vi "UHR-Fleezers Control (host) - 12.0.vi"() -> ()   [LabVIEW 2012] (continued)
                n291 = Divide "X half step offset"(x=w508, y=2.0) -> (x/y=w516:dbl)
                n292 = Divide "X V/pix"(x=w508, y=w519) -> (x/y=w518:dbl)
                n293 = Multiply(x=w508, y=w513) -> (x*y=w525:dbl)
                n294 = Compound Arithmetic op=ADD(w523, w530, w529) -> (w500:dbl)
                "Pointer Y (V)" <- w500
                n295 = Multiply(x=w518, y=w512) -> (x*y=w527:dbl)
                n296 = Negate(x=w516) -> (-x=w515:dbl)
                n297 = local read "Initial X"() -> (w528:dbl)
                n298 = Negate(x=w527) -> (-x=w526:dbl)
                n299 = Compound Arithmetic op=ADD(w515, w525, w528, w526) -> (w501:dbl)
                "Pointer X (V)" <- w501
                n300 = case shown="True" "Set High F Confocal Spot (X-Y)" {
                  tunnel: w501 -> [_ w531]
                  tunnel: w500 -> [_ w532]
                  frame False {
                  }
                  frame True {
                    "Confocal Y 2 (V)" <- w532
                    "Confocal X 2 (V)" <- w531
                  }
                }
                n301 = Or(x="Set X Only", y="Set Confocal Spot (X-Y)") -> (x .or. y?=w504:bool)
                n302 = Or(x="Set Confocal Spot (X-Y)", y="Set Y Only") -> (x .or. y?=w503:bool)
                n303 = case shown="True" w504 {
                  tunnel: w501 -> [_ w533]
                  frame False {
                  }
                  frame True {
                    n304 = property on="AO2" class="Slide (strict)"("Val(Sgnl)"=w533) -> ()  [unwired: 2 in, 2 out]
                    "Confocal X 1 (V)" <- w533
                  }
                }
                n305 = case shown="True" w503 {
                  tunnel: w500 -> [_ w534]
                  frame False {
                  }
                  frame True {
                    n306 = property on="AO1" class="Slide (strict)"("Val(Sgnl)"=w534) -> ()  [unwired: 2 in, 2 out]
                    "Confocal Y 1 (V)" <- w534
                  }
                }
                n307 = local write "Set High F Confocal Spot (X-Y)"(w499) -> ()
                n308 = local write "Set Confocal Spot (X-Y)"(w499) -> ()
                n309 = local write "Set X Only"(w499) -> ()
                n310 = local write "Set Y Only"(w499) -> ()
              }
            }
          }
          frame 3 {
            n311 = local read "BD 2 Frequency 1 (MHz)"() -> (w535:dbl)
            n312 = local read "BD 1 Frequency 1 (MHz)"() -> (w536:dbl)
            n313 = local write "Manipulating Trap"(TRUE ("Manipulating Trap")) -> ()
            n314 = local write "Coords"(T7 {"Horizontal"=0, "Vertical"=0} ("Coords")) -> ()
            n315 = while {
              tunnel: w541 -> [w546]
              tunnel: w539 -> [w545]
              tunnel: w537 -> [w544]
              tunnel: w536 -> [w543]
              tunnel: w535 -> [w542]
              stop <- w547 stop-if-true
              n316 = event shown="[0] \"Pane\": Mouse Move" {
                selector: _ -> [_ _]
                dyn-events: _ -> [_ _]
                timeout: _ -> [_ _]
                tunnel: ["Force Manip Abort" w611] -> w547
                tunnel: w546 -> [w554 _]
                tunnel: w545 -> [w552 _]
                tunnel: w544 -> [w551 _]
                tunnel: w543 -> [w550 _]
                tunnel: w542 -> [w549 _]
                event Mouse Move {
                  n317 = event-data() -> ("Time"=w555:u32, "Coords"=w556:T7)  [unwired: 3 out]
                  n318 = Less?(x=w555, y=w554) -> (x < y?=w553:bool)
                  n319 = case "Makes sure old motion events prior to mouse click aren't used" shown="False" w553 {
                    tunnel: w556 -> [w598 _]
                    tunnel: w552 -> [w599 _]
                    tunnel: w551 -> [w576 _]
                    tunnel: w550 -> [w572 _]
                    tunnel: w549 -> [w571 _]
                    frame False {
                      n320 = Subtract(x=w598, y=w599) -> (x-y=w597:T7)
                      "Coords" <- w597
                      n321 = local read "Y RF Frequency Limits (MHz)"() -> (w557:T16)
                      n322 = To Double Precision Float(number=w597) -> (double precision float=w596:cluster{"Horizontal":dbl, "Vertical":dbl})
                      n323 = Multiply(x=cluster{"Horizontal":dbl, "Vertical":dbl} {"Horizontal"=-1.0, "Vertical"=1.0}, y="Manipulation Scaling") -> (x*y=w592:cluster{"Horizontal":dbl, "Vertical":dbl})
                      n324 = local read "X RF Frequency Limits (MHz)"() -> (w558:T16)
                      n325 = Multiply(x=w596, y=w592) -> (x*y=w594:cluster{"Horizontal":dbl, "Vertical":dbl})
                      n326 = Unbundle By Name(w594) -> ("Horizontal"=w589:dbl, "Vertical"=w593:dbl)
                      n327 = Unbundle By Name(w557) -> ("Maximum"=w560:dbl, "Minimum"=w559:dbl)
                      n328 = Boolean To (0,1)(Boolean="Manip. X?") -> (0, 1=w587:i16)
                      n329 = Boolean To (0,1)(Boolean="Manip. Y?") -> (0, 1=w584:i16)
                      n330 = local read "BD 1 Frequency 2 (MHz)"() -> (w574:dbl)
                      n331 = Multiply(x=w593, y=w584) -> (x*y=w586:dbl)
                      n332 = Multiply(x=w587, y=w589) -> (x*y=w590:dbl)
                      n333 = local read "BD 2 Frequency 2 (MHz)"() -> (w573:dbl)
                      n334 = Unbundle By Name(w558) -> ("Maximum"=w562:dbl, "Minimum"=w561:dbl)
                      n335 = Add(x=w571, y=w586) -> (x+y=w564:dbl)
                      n336 = Add(x=w572, y=w590) -> (x+y=w566:dbl)
                      n337 = In Range and Coerce(upper limit=w562, x=w566, lower limit=w561) -> (coerced(x)=w565:dbl)  [unwired: 1 out]
                      n338 = In Range and Coerce(upper limit=w560, x=w564, lower limit=w559) -> (coerced(x)=w563:dbl)  [unwired: 1 out]
                      n339 = Subtract(x=w565, y=w574) -> (x-y=w583:dbl)
                      n340 = Subtract(x=w563, y=w573) -> (x-y=w582:dbl)
                      n341 = Square(x=w583) -> (x^2=w581:dbl)
                      n342 = Square(x=w582) -> (x^2=w580:dbl)
                      n343 = Add(x=w581, y=w580) -> (x+y=w579:dbl)
                      n344 = Square Root(x=w579) -> (sqrt(x)=w575:dbl)
                      n345 = In Range and Coerce(upper limit="Limit Max (MHz)", x=w575, lower limit="Limit Min (MHz)") -> (In Range?=w568:bool)  [unwired: 1 out]
                      n346 = Not(x="Limits Enable") -> (.not. x?=w567:bool)
                      n347 = Or(x=w568, y=w567) -> (x .or. y?=w569:bool)
                      n348 = case shown="True" w569 {
                        tunnel: w576 -> [_ w609]
                        tunnel: w575 -> [_ w600]
                        tunnel: w565 -> [_ w607]
                        tunnel: w574 -> [_ w606]
                        tunnel: w563 -> [_ w605]
                        tunnel: w573 -> [_ w604]
                        tunnel: w558 -> [_ w602]
                        tunnel: w557 -> [_ w601]
                        frame False {
                        }
                        frame True {
                          n349 = local read "BD 1 Frequency 3 (MHz)"() -> (w608:dbl)
                          n350 = local read "BD 2 Frequency 3 (MHz)"() -> (w603:dbl)
                          n351 = local write "Trap Delta (MHz)"(w600) -> ()
                          n352 = call "set RF board frequency - interlace.vi"("Board 2 Frequency Limits"=w601, "Board 1 Frequency Limits"=w602, "FPGA VI Reference In"=w609, "Board 2 Frequency 3 (MHz)"=w603, "Board 1 Frequency 3 (MHz)"=w608, "Board 2 Frequency 2 (MHz)"=w604, "Board 2 Frequency 1 (MHz)"=w605, "Board 1 Frequency 2 (MHz)"=w606, "Board 1 Frequency 1  (MHz)"=w607) -> ()  [unwired: 1 in, 2 out]
                          n353 = local write "BD 2 Frequency 1 (MHz)"(w605) -> ()
                          n354 = local write "BD 1 Frequency 1 (MHz)"(w607) -> ()
                        }
                      }
                    }
                    frame True {
                    }
                  }
                }
                event Mouse Up {
                  n355 = event-data() -> ("Button"=w610:u16)  [unwired: 8 out]
                  n356 = case shown="3" w610 {
                    tunnel: [FALSE TRUE] -> w611
                    frame 0, Default {
                    }
                    frame 3 {
                      n357 = local read "Trap Delta (MHz)"() -> (w613:dbl)
                      n358 = property on="Initial delta (MHz)" class="DigNum (strict)"("Val(Sgnl)"=w613) -> ()  [unwired: 2 in, 2 out]
                      n359 = local write "Manipulating Trap"(FALSE ("Manipulating Trap")) -> ()
                    }
                  }
                }
              }
            }
          }
        }
      }
      event Mouse Move {
        n360 = event-data() -> ()  [unwired: 6 out]
      }
    }
    n361 = local read "Stop All"() -> (w429:bool)
    n362 = node-c288() -> ()  [unwired: 2 out]
  }
  n363 = timed-loop "Run Scripts, including: stage motion" {
    tunnel: w89 -> [w622]
    tunnel: w88 -> [w623]
    tunnel: [w623] -> w87
    tunnel: [w622] -> w86
    timing: w84 -> [_]
    timing-out: [_] -> w83
    tunnel: w69 -> [w621]
    tunnel: w70 -> [w620]
    tunnel: w10 -> [w617]
    tunnel: w9 -> [w616]
    tunnel: w8 -> [w618]
    tunnel: w7 -> [w619]
    stop <- w624 stop-if-true
    n364 = node-c288() -> ()  [unwired: 1 in, 1 out]
    n365 = event shown="[12] \"Force FB Data Script\": Value Change" {
      selector: _ -> [_ _ _ _ _ _ _ _ _ _ _ _ _ _ _ _ _ _ _]
      dyn-events: _ -> [_ _ _ _ _ _ _ _ _ _ _ _ _ _ _ _ _ _ _]
      timeout: _ -> [_ _ _ _ _ _ _ _ _ _ _ _ _ _ _ _ _ _ _]
      tunnel: ["Set Position" "Move to Position" _ _ "Read Harvard" _ _ _ _ _ _ "Got ADig bead" "Force FB Data\nScript" _ "Got DNA bead" "Take Stepping Data" _ "Take Detection Laser\nImage" _] -> _
      tunnel: [_ _ _ _ _ _ _ _ _ _ _ _ _ _ _ _ _ _ w1241] -> w624
      tunnel: w622 -> [w642 w650 w663 w693 _ w738 w778 w859 w888 w1020 w1046 _ w1082 _ _ _ _ _ _]
      tunnel: w623 -> [w643 w651 w664 w694 _ w739 w779 w860 w889 w1021 w1047 _ w1083 _ _ _ _ _ _]
      tunnel: w621 -> [_ _ _ _ w723 _ _ _ _ _ _ _ _ _ _ _ _ _ _]
      tunnel: w620 -> [_ _ _ _ w722 _ _ _ _ _ _ _ _ _ _ _ _ _ _]
      tunnel: w619 -> [_ _ _ _ _ _ _ _ _ _ _ _ _ _ _ _ _ _ _]
      tunnel: w618 -> [_ _ _ _ _ _ _ _ _ _ _ _ _ _ _ _ _ _ _]
      tunnel: w617 -> [_ _ _ _ _ _ _ _ _ _ _ _ _ _ _ _ _ _ _]
      tunnel: w616 -> [_ _ _ _ _ _ _ _ _ _ _ _ _ _ _ _ _ _ _]
      event "Set Position", "Set Position 2", "Set Position 3", "Set Position 4", "Set Position 5", "Set Position 1": Value Change {
        n366 = event-data() -> ()  [unwired: 1 in, 5 out]
        n367 = Build Array("Set Position 1", "Set Position 2", "Set Position 3", "Set Position 4", "Set Position 5") -> (w641:bool[])
        n368 = Boolean Array To Number(Boolean array=w641) -> (number=w640:u32)
        n369 = Logarithm Base 2(1:w640) -> (0:w632:dbl)
        n370 = call "Read Stage Position.vi"("error in"=w642, "VISA resource name in"=w643) -> ("Current Position"=w647:cluster{dbl, dbl, dbl}, "error out"=w646:errorcluster)  [unwired: 2 out]
        n371 = Decrement(x="Position") -> (x-1=w630:dbl)
        n372 = Greater Or Equal?(x=w632, y=0.0) -> (x >= y?=w633:bool)
        n373 = Cluster To Array(cluster=w647) -> (array=w644:dbl[])
        n374 = local write "Stage Control Serial Error"(w646) -> ()
        n375 = Select(t=w632, s=w633, f=w630) -> (s? t:f=w629:dbl)
        n376 = Increment(x=w629) -> (x+1=w628:dbl)
        n377 = Build Array (concatenate)(w628, w644) -> (w627:dbl[])
        n378 = Replace Array Subset(array="Saved Stage Positions", new element=w627, index (row)=w629) -> (w645:dbl[][])  [unwired: 1 in]
        n379 = local write "Saved Stage Positions"(w645) -> ()
      }
      event "Move to Position": Value Change {
        n380 = event-data() -> ()  [unwired: 1 in, 5 out]
        n381 = flat-sequence {
          tunnel: w651 -> [w655]
          tunnel: w650 -> [w654]
          frame #0 {
            n382 = local read "Saved Stage Positions"() -> (w657:dbl[][])
            n383 = local read "Position"() -> (w656:dbl)
            n384 = local write "Stage Moving"(TRUE ("Stage Moving")) -> ()
            n385 = call "move to saved stage position.vi"("error in"=w654, "Stage VISA resource name in"=w655, "Position"=w656, "Saved Stage Positions"=w657) -> ("error out"=w653:errorcluster)  [unwired: 1 out]
            n386 = local write "Stage Control Serial Error"(w653) -> ()
          }
          frame #1 {
            n387 = call <vilib>:"Beep.vi"() -> ()  [unwired: 3 in, 9 out]
            n388 = local write "Stage Moving"(FALSE ("Stage Moving")) -> ()
          }
        }
      }
      event "Move Cap. 1 (DNA Bottom)": Value Change {
        n389 = event-data() -> ()  [unwired: 1 in, 5 out]
        n390 = local write "Move Cap. 1 (DNA Bottom)"(FALSE ("Move Cap. 1 (DNA Right)")) -> ()
        n391 = flat-sequence {
          tunnel: w663 -> [w666]
          tunnel: w664 -> [w667]
          tunnel: [w667] -> w661
          tunnel: [w666] -> w660
          tunnel: w661 -> [w669]
          tunnel: w660 -> [w668]
          frame #0 {
            n392 = property on="Sample Channel\nFlow" class="Bool (strict)"("Val(Sgnl)"="Cap 1 Samp Flow ON") -> ()  [unwired: 2 in, 2 out]
          }
          frame #1 {
            n393 = local read "Saved Stage Positions"() -> (w679:dbl[][])
            n394 = local write "Stage Moving"(TRUE ("Stage Moving")) -> ()
            n395 = Array Subset(array=w679, index (row)=0 ("index"), length (row)=1 ("length"), index (col)=1 ("index"), length (col)=3 ("length")) -> (w676:dbl[][])
            n396 = Reshape Array(w676, 3 ("dimension size")) -> (w674:dbl[])
            n397 = Array To Cluster(array=w674) -> (cluster=w673:cluster{"[0]":dbl, "[1]":dbl, "[2]":dbl})
            n398 = call "Set Stage Position.vi"("Position"=w673, "error in"=w668, "VISA resource name in"=w669) -> ("error out"=w672:errorcluster)  [unwired: 2 out]
            n399 = local write "Stage Control Serial Error"(w672) -> ()
          }
          frame #2 {
            n400 = local write "Stage Moving"(FALSE ("Stage Moving")) -> ()
            n401 = case shown="True" "Cap 1 Flow ON" {
              frame False {
              }
              frame True {
                n402 = property on="Inject Pump 1" class="Bool (strict)"("Val(Sgnl)"=TRUE ("Value (Signaling)")) -> ()  [unwired: 2 in, 2 out]
              }
            }
            n403 = call <vilib>:"Beep.vi"() -> ()  [unwired: 3 in, 9 out]
          }
          frame #3 {
            n404 = property on="Sample Channel\nFlow" class="Bool (strict)"("Val(Sgnl)"=FALSE ("Value (Signaling)")) -> ()  [unwired: 2 in, 2 out]
            n405 = local read "Cap. 2 BD T1?\n(ADig T1, DNA T2)"() -> (w686:bool)
            n406 = case shown="True" w686 {
              tunnel: "Cap 1 T ON" -> [w688 w689]
              frame False {
                n407 = property on="Trap 1 (ON/OFF)" class="Bool (strict)"("Val(Sgnl)"=w688) -> ()  [unwired: 2 in, 2 out]
              }
              frame True {
                n408 = property on="Trap 2 (ON/OFF)" class="Bool (strict)"("Val(Sgnl)"=w689) -> ()  [unwired: 2 in, 2 out]
              }
            }
            n409 = property on="Got DNA bead" class="Bool"("Key Focus"=TRUE) -> ()  [unwired: 2 in, 2 out]
          }
        }
      }
      event "Move Cap. 2 (ADig Top)": Value Change {
        n410 = event-data() -> ()  [unwired: 1 in, 5 out]
        n411 = local write "Move Cap. 2 (ADig Top)"(FALSE ("Move Cap. 2 (ADig Left)")) -> ()
        n412 = flat-sequence {
          tunnel: w693 -> [w696]
          tunnel: w694 -> [w697]
          tunnel: [w697] -> w691
          tunnel: [w696] -> w690
          tunnel: w691 -> [w700]
          tunnel: w690 -> [w699]
          frame #0 {
            n413 = property on="Sample Channel\nFlow" class="Bool (strict)"("Val(Sgnl)"="Cap 2 Samp Flow ON") -> ()  [unwired: 2 in, 2 out]
          }
          frame #1 {
            w698 = FALSE ("Value (Signaling)")
            n414 = local read "Saved Stage Positions"() -> (w710:dbl[][])
            n415 = local write "Stage Moving"(TRUE ("Stage Moving")) -> ()
            n416 = Array Subset(array=w710, index (row)=1 ("index"), length (row)=1 ("length"), index (col)=1 ("index"), length (col)=3 ("length")) -> (w707:dbl[][])
            n417 = Reshape Array(w707, 3 ("dimension size")) -> (w705:dbl[])
            n418 = property on="Trap 1 (ON/OFF)" class="Bool (strict)"("Val(Sgnl)"=w698) -> ()  [unwired: 2 in, 2 out]
            n419 = property on="Trap 1 (ON/OFF)" class="Bool (strict)"("Val(Sgnl)"=w698) -> ()  [unwired: 2 in, 2 out]
            n420 = Array To Cluster(array=w705) -> (cluster=w704:cluster{"[0]":dbl, "[1]":dbl, "[2]":dbl})
            n421 = call "Set Stage Position.vi"("Position"=w704, "error in"=w699, "VISA resource name in"=w700) -> ("error out"=w703:errorcluster)  [unwired: 2 out]
            n422 = local write "Stage Control Serial Error"(w703) -> ()
          }
          frame #2 {
            n423 = local write "Stage Moving"(FALSE ("Stage Moving")) -> ()
            n424 = call <vilib>:"Beep.vi"() -> ()  [unwired: 3 in, 9 out]
            n425 = case shown="True" "Cap 2 Flow ON" {
              frame False {
              }
              frame True {
                n426 = property on="Inject Pump 3" class="Bool (strict)"("Val(Sgnl)"=TRUE ("Value (Signaling)")) -> ()  [unwired: 2 in, 2 out]
              }
            }
          }
          frame #3 {
            n427 = property on="Sample Channel\nFlow" class="Bool (strict)"("Val(Sgnl)"=FALSE ("Value (Signaling)")) -> ()  [unwired: 2 in, 2 out]
            n428 = case shown="False" "Cap. 2 BD T1?\n(ADig T1, DNA T2)" {
              tunnel: "Cap 2 T ON" -> [w719 w720]
              frame False {
                n429 = property on="Trap 2 (ON/OFF)" class="Bool (strict)"("Val(Sgnl)"=w719) -> ()  [unwired: 2 in, 2 out]
              }
              frame True {
                n430 = property on="Trap 1 (ON/OFF)" class="Bool (strict)"("Val(Sgnl)"=w720) -> ()  [unwired: 2 in, 2 out]
              }
            }
            n431 = property on="Got ADig bead" class="Bool"("Key Focus"=TRUE) -> ()  [unwired: 2 in, 2 out]
          }
        }
      }
      event "Read Harvard": Value Change {
        n432 = event-data() -> ()  [unwired: 1 in, 5 out]
        n433 = Concatenate Strings("write buffer", "\r") -> (w725:string)
        n434 = VISA Write(VISA resource name=w723, write buffer=w725, error in (no error)=w722) -> (VISA resource name out=w734:refnum<visa-resource-name>, error out=w733:errorcluster)  [unwired: 1 out]
        n435 = stacked-sequence {
          tunnel: [w737] -> w732
          tunnel: w734 -> [w737]
          tunnel: w733 -> [w736]
          tunnel: [w736] -> w727
          frame #0 {
            n436 = Wait (ms)(milliseconds to wait=50) -> ()  [unwired: 1 out]
          }
        }
        n437 = property class="Instr"(reference=w732, error in=w727) -> (reference out=w731:refnum<visa-resource-name>, error out=w729:errorcluster, "Serial Settings:Number of Bytes at Serial Port"=w730:u32)
        "Serial Settings:Number of Bytes at Serial Port" <- w730
        n438 = VISA Read(VISA resource name=w731, byte count=w730, error in (no error)=w729) -> (read buffer=w728:string)  [unwired: 3 out]
        "read buffer" <- w728
        n439 = Fract/Exp String To Number(string=w728) -> ()  [unwired: 5 out]
      }
      event "+z", "-z": Value Change {
        n440 = event-data() -> ()  [unwired: 1 in, 5 out]
        n441 = flat-sequence {
          tunnel: w738 -> [w760]
          tunnel: w739 -> [w740]
          frame #0 {
            n442 = call "Read Stage Position.vi"("error in"=w760, "VISA resource name in"=w740) -> ("Current Position"=w745:cluster{dbl, dbl, dbl}, "error out"=w758:errorcluster, "VISA resource name out"=w759:refnum<visa-resource-name>)  [unwired: 1 out]
            n443 = local read "Saved Stage Positions"() -> (w769:dbl[][])
            n444 = Divide(x="z nudge increment (um)", y=1000.0) -> (x/y=w757:dbl)
            n445 = Boolean To (0,1)(Boolean="+z") -> (0, 1=w749:i16)
            n446 = Boolean To (0,1)(Boolean="-z") -> (0, 1=w750:i16)
            n447 = Array Subset(array=w769, index (row)=1 ("index"), length (row)=1 ("length"), index (col)=1 ("index"), length (col)=3 ("length")) -> (w766:dbl[][])
            n448 = Multiply(x=w749, y=w757) -> (x*y=w753:dbl)
            n449 = Multiply(x=w750, y=w757) -> (x*y=w751:dbl)
            n450 = Unbundle(w745) -> (w743:dbl, w742:dbl, w746:dbl)
            n451 = Negate(x=w751) -> (-x=w752:dbl)
            n452 = Reshape Array(w766, 3 ("dimension size")) -> (w764:dbl[])
            n453 = Add(x=w753, y=w752) -> (x+y=w754:dbl)
            n454 = Array To Cluster(array=w764) -> ()  [unwired: 1 out]
            n455 = Add(x=w754, y=w746) -> (x+y=w744:dbl)
            n456 = Bundle(cluster=w745, w743, w742, w744) -> (w741:cluster{dbl, dbl, dbl})
            n457 = call "Set Stage Position.vi"("Position"=w741, "error in"=w758, "VISA resource name in"=w759) -> ("error out"=w763:errorcluster)  [unwired: 2 out]
            n458 = local write "Stage Moving"(TRUE ("Stage Moving")) -> ()
            n459 = local write "Stage Control Serial Error"(w763) -> ()
          }
          frame #1 {
            n460 = local write "Stage Moving"(FALSE ("Stage Moving")) -> ()
            n461 = call <vilib>:"Beep.vi"() -> ()  [unwired: 3 in, 9 out]
          }
        }
      }
      event "Cal/Data Acq. Spot": Value Change {
        n462 = event-data() -> ()  [unwired: 1 in, 5 out]
        n463 = flat-sequence {
          tunnel: w778 -> [w782]
          tunnel: w779 -> [w783]
          tunnel: [w783] -> w775
          tunnel: [w782] -> w774
          tunnel: w775 -> [w788]
          tunnel: w774 -> [w787]
          tunnel: ["Cal @ (MHz)"] -> w772
          tunnel: [w792] -> w776
          tunnel: w772 -> [w792]
          tunnel: w776 -> [w801]
          tunnel: ["W/ Offset 1"] -> w773
          tunnel: w776 -> [w822]
          tunnel: w773 -> [w820]
          frame #0 {
            n464 = property on="Sample Channel\nFlow" class="Bool (strict)"("Val(Sgnl)"="Daq spot flow on") -> ()  [unwired: 2 in, 2 out]
            n465 = Wait (ms)(milliseconds to wait=u32 250) -> ()  [unwired: 1 out]
          }
          frame #1 {
            n466 = local read "Saved Stage Positions"() -> (w785:dbl[][])
            n467 = property on="Trap Delta (MHz)" class="DigNum (strict)"("Val(Sgnl)"="Cal @ (MHz)") -> ()  [unwired: 2 in, 2 out]
            n468 = local write "Stage Moving"(TRUE ("Stage Moving")) -> ()
            n469 = call "move to saved stage position.vi"("error in"=w787, "Stage VISA resource name in"=w788, "Position"="Cal Stage Position", "Saved Stage Positions"=w785) -> ("error out"=w786:errorcluster)  [unwired: 1 out]
            n470 = local write "Stage Control Serial Error"(w786) -> ()
          }
          frame #2 {
            n471 = local write "Stage Moving"(FALSE ("Stage Moving")) -> ()
            n472 = property on="Sample Channel\nFlow" class="Bool (strict)"("Val(Sgnl)"="Flow ON during cal?") -> ()  [unwired: 2 in, 2 out]
            n473 = call <vilib>:"Beep.vi"() -> ()  [unwired: 3 in, 9 out]
          }
          frame #3 {
            n474 = Wait (ms)(milliseconds to wait=u32 1000) -> ()  [unwired: 1 out]
          }
          frame #4 {
            n475 = property on="Save Calibration" class="Bool (strict)"("Val(Sgnl)"=TRUE ("Value (Signaling)")) -> ()  [unwired: 2 in, 2 out]
          }
          frame #5 {
            n476 = Wait (ms)(milliseconds to wait=u32 2000) -> ()  [unwired: 1 out]
          }
          frame #6 {
            # "Check to see if \nsaving done"
            n477 = while {
              stop <- w797 stop-if-true
              n478 = local read "Saving..."() -> (w798:bool)
              n479 = Wait (ms)(milliseconds to wait=u32 100) -> ()  [unwired: 1 out]
              n480 = Not(x=w798) -> (.not. x?=w797:bool)
            }
          }
          frame #7 {
            n481 = case shown="True" "W/ Offset 1" {
              tunnel: w801 -> [_ w802]
              frame False {
              }
              frame True {
                n482 = stacked-sequence {
                  tunnel: w802 -> [_ _ _ _ _ _ _ w819]
                  frame #0 {
                    n483 = property on="Trap Delta (MHz)" class="DigNum (strict)"("Val(Sgnl)"="Offset 1 Start (MHz)") -> ()  [unwired: 2 in, 2 out]
                    n484 = Replace Array Subset(array=u32[] [0] ("Index Values"), new element="Offset 1 Set", index=0) -> (w803:u32[])
                    n485 = property on="Saved AOD Raster Scan Parameter Sets" class="Arr (strict)"("Index Values"=w803) -> ()  [unwired: 2 in, 2 out]
                  }
                  frame #1 {
                    n486 = Wait (ms)(milliseconds to wait=u32 200) -> ()  [unwired: 1 out]
                  }
                  frame #2 {
                    n487 = property on="Load parameters" class="Bool (strict)"("Val(Sgnl)"=TRUE ("Value (Signaling)")) -> ()  [unwired: 2 in, 2 out]
                  }
                  frame #3 {
                    n488 = Wait (ms)(milliseconds to wait=u32 200) -> ()  [unwired: 1 out]
                  }
                  frame #4 {
                    n489 = property on="Trap Raster Scan" class="Bool (strict)"("Val(Sgnl)"=TRUE ("Value (Signaling)")) -> ()  [unwired: 2 in, 2 out]
                  }
                  frame #5 {
                    n490 = Wait (ms)(milliseconds to wait=u32 2000) -> ()  [unwired: 1 out]
                  }
                  frame #6 {
                    n491 = while {
                      stop <- w816 stop-if-true
                      n492 = local read "Raster Scanning..."() -> (w818:bool)
                      n493 = local read "Saving..."() -> (w814:bool)
                      n494 = Wait (ms)(milliseconds to wait=u32 100) -> ()  [unwired: 1 out]
                      n495 = Not(x=w814) -> (.not. x?=w813:bool)
                      n496 = Not(x=w818) -> (.not. x?=w815:bool)
                      n497 = And(x=w815, y=w813) -> (x .and. y?=w816:bool)
                    }
                  }
                  frame #7 {
                    n498 = property on="Trap Delta (MHz)" class="DigNum (strict)"("Val(Sgnl)"=w819) -> ()  [unwired: 2 in, 2 out]
                  }
                }
              }
            }
          }
          frame #8 {
            n499 = local read "Save ave N"() -> (w821:dbl)
            n500 = case shown="False" "W/ Offset 2" {
              tunnel: w822 -> [_ w829]
              tunnel: w821 -> [_ w828]
              tunnel: w820 -> [w824 _]
              frame False {
                n501 = case shown="False" w824 {
                  frame False {
                    n502 = Multiply(x="Cal read wait (s)", y=u32 1000 ("milliseconds to wait")) -> (x*y=w826:u32)
                    n503 = Wait (ms)(milliseconds to wait=w826) -> ()  [unwired: 1 out]
                  }
                  frame True {
                  }
                }
              }
              frame True {
                n504 = stacked-sequence {
                  tunnel: w829 -> [_ _ _ _ _ _ _ _ _ w850 _ _]
                  tunnel: w828 -> [_ _ _ _ _ _ _ _ _ w848 _ _]
                  frame #0 {
                    n505 = property on="Save ave N" class="DigNum (strict)"("Val(Sgnl)"=1.0 ("Value (Signaling)")) -> ()  [unwired: 2 in, 2 out]
                  }
                  frame #1 {
                    n506 = Wait (ms)(milliseconds to wait=u32 500) -> ()  [unwired: 1 out]
                  }
                  frame #2 {
                    n507 = property on="Trap Delta (MHz)" class="DigNum (strict)"("Val(Sgnl)"="Offset 2 Start (MHz)") -> ()  [unwired: 2 in, 2 out]
                    n508 = Replace Array Subset(array=u32[] [0] ("Index Values"), new element="Offset 2 Set", index=0) -> (w834:u32[])
                    n509 = property on="Saved AOD Raster Scan Parameter Sets" class="Arr (strict)"("Index Values"=w834) -> ()  [unwired: 2 in, 2 out]
                  }
                  frame #3 {
                    n510 = Wait (ms)(milliseconds to wait=u32 500) -> ()  [unwired: 1 out]
                  }
                  frame #4 {
                    n511 = property on="Load parameters" class="Bool (strict)"("Val(Sgnl)"=TRUE ("Value (Signaling)")) -> ()  [unwired: 2 in, 2 out]
                  }
                  frame #5 {
                    n512 = Wait (ms)(milliseconds to wait=u32 500) -> ()  [unwired: 1 out]
                  }
                  frame #6 {
                    n513 = property on="Trap Raster Scan" class="Bool (strict)"("Val(Sgnl)"=TRUE ("Value (Signaling)")) -> ()  [unwired: 2 in, 2 out]
                  }
                  frame #7 {
                    n514 = Wait (ms)(milliseconds to wait=u32 2000) -> ()  [unwired: 1 out]
                  }
                  frame #8 {
                    n515 = while {
                      stop <- w843 stop-if-true
                      n516 = local read "Raster Scanning..."() -> (w846:bool)
                      n517 = local read "Saving..."() -> (w844:bool)
                      n518 = Wait (ms)(milliseconds to wait=u32 100) -> ()  [unwired: 1 out]
                      n519 = Not(x=w844) -> (.not. x?=w842:bool)
                      n520 = Not(x=w846) -> (.not. x?=w845:bool)
                      n521 = And(x=w845, y=w842) -> (x .and. y?=w843:bool)
                    }
                  }
                  frame #9 {
                    n522 = property on="Trap Delta (MHz)" class="DigNum (strict)"("Val(Sgnl)"=w850) -> ()  [unwired: 2 in, 2 out]
                    n523 = property on="Saved AOD Raster Scan Parameter Sets" class="Arr (strict)"("Index Values"=u32[] [0]) -> ()  [unwired: 2 in, 2 out]
                    n524 = property on="Save ave N" class="DigNum (strict)"("Val(Sgnl)"=w848) -> ()  [unwired: 2 in, 2 out]
                  }
                  frame #10 {
                    n525 = Wait (ms)(milliseconds to wait=u32 500) -> ()  [unwired: 1 out]
                  }
                  frame #11 {
                    n526 = property on="Load parameters" class="Bool (strict)"("Val(Sgnl)"=TRUE ("Value (Signaling)")) -> ()  [unwired: 2 in, 2 out]
                  }
                }
              }
            }
          }
          frame #9 {
            n527 = property on="Read Cal" class="Bool (strict)"("Val(Sgnl)"=TRUE ("Value (Signaling)")) -> ()  [unwired: 2 in, 2 out]
          }
          frame #10 {
            n528 = Wait (ms)(milliseconds to wait=u32 1000) -> ()  [unwired: 1 out]
          }
          frame #11 {
            n529 = property on="Fish for Tether" class="Bool (strict)"("Val(Sgnl)"=TRUE ("Value (Signaling)")) -> ()  [unwired: 2 in, 2 out]
          }
        }
        n530 = local write "Cal/Data Acq. Spot"(FALSE ("Cal/Data Acq. Spot")) -> ()
      }
      event "Dump Beads": Value Change {
        n531 = event-data() -> ()  [unwired: 1 in, 5 out]
        n532 = flat-sequence {
          tunnel: ["Dump spot flow on?"] -> w856
          tunnel: [w867] -> w857
          tunnel: w856 -> [w867]
          tunnel: w860 -> [w872]
          tunnel: w859 -> [w871]
          tunnel: [w869] -> w858
          tunnel: w857 -> [w869]
          tunnel: w858 -> [w882]
          frame #0 {
            w861 = FALSE ("Value (Signaling)")
            n533 = local read "Saving..."() -> (w863:bool)
            n534 = local write "Dump Beads"(FALSE ("Dump Beads")) -> ()
            n535 = property on="Inject Pump 3" class="Bool (strict)"("Val(Sgnl)"=w861) -> ()  [unwired: 2 in, 2 out]
            n536 = property on="Inject Pump 1" class="Bool (strict)"("Val(Sgnl)"=w861) -> ()  [unwired: 2 in, 2 out]
            n537 = local write "Stop Saving"(w863) -> ()
          }
          frame #1 {
            w864 = FALSE ("Fl. Triggered...")
            n538 = case shown="True" "Dump spot flow on?" {
              frame False {
              }
              frame True {
                n539 = property on="Sample Channel\nFlow" class="Bool (strict)"("Val(Sgnl)"=TRUE ("Stage Moving")) -> ()  [unwired: 2 in, 2 out]
              }
            }
            n540 = local write "Fl. Triggered..."(w864) -> ()
            n541 = local write "Tether"(w864) -> ()
            n542 = property on="Green Laser ON/Interlacing" class="Bool (strict)"("Val(Sgnl)"=w864) -> ()  [unwired: 2 in, 2 out]
            n543 = property on="Trap Pos. FB ON" class="Bool (strict)"("Val(Sgnl)"=w864) -> ()  [unwired: 2 in, 2 out]
            n544 = property on="Trap Trig. Fl." class="Bool (strict)"("Val(Sgnl)"=w864) -> ()  [unwired: 2 in, 2 out]
            n545 = property on="Fl. Triggered..." class="Bool (strict)"("Val(Sgnl)"=w864) -> ()  [unwired: 2 in, 2 out]
            n546 = property on="Dip for Protein" class="Bool (strict)"("Val(Sgnl)"=w864) -> ()  [unwired: 2 in, 2 out]
            n547 = property on="Pause dwell" class="Bool (strict)"("Val(Sgnl)"=w864) -> ()  [unwired: 2 in, 2 out]
          }
          frame #2 {
            n548 = property on="Trap Pos. FB Offset Factor" class="DigNum (strict)"("Val(Sgnl)"=i64 0 ("Value (Signaling)")) -> ()  [unwired: 2 in, 2 out]
          }
          frame #3 {
            n549 = local read "Saved Stage Positions"() -> (w873:dbl[][])
            n550 = local write "Stage Moving"(TRUE ("Stage Moving")) -> ()
            n551 = Array Subset(array=w873, index (row)=3 ("index"), length (row)=1 ("length"), index (col)=1 ("index"), length (col)=3 ("length")) -> (w878:dbl[][])
            n552 = Reshape Array(w878, 3 ("dimension size")) -> (w876:dbl[])
            n553 = Array To Cluster(array=w876) -> (cluster=w875:cluster{"[0]":dbl, "[1]":dbl, "[2]":dbl})
            n554 = call "Set Stage Position.vi"("Position"=w875, "error in"=w871, "VISA resource name in"=w872) -> ()  [unwired: 3 out]
          }
          frame #4 {
            w883 = FALSE ("Value (Signaling)")
            n555 = case shown="True" w882 {
              frame False {
              }
              frame True {
                n556 = property on="Sample Channel\nFlow" class="Bool (strict)"("Val(Sgnl)"=FALSE ("Stage Moving")) -> ()  [unwired: 2 in, 2 out]
              }
            }
            n557 = property on="Trap 1 (ON/OFF)" class="Bool (strict)"("Val(Sgnl)"=w883) -> ()  [unwired: 2 in, 2 out]
            n558 = property on="Trap 2 (ON/OFF)" class="Bool (strict)"("Val(Sgnl)"=w883) -> ()  [unwired: 2 in, 2 out]
            n559 = call <vilib>:"Beep.vi"() -> ()  [unwired: 3 in, 9 out]
          }
          frame #5 {
            n560 = property on="Move Cap. 2 (ADig Top)" class="Bool (strict)"("Val(Sgnl)"=TRUE ("Value (Signaling)")) -> ()  [unwired: 2 in, 2 out]
            n561 = property on="Tab Control" class="TabCtl (strict)"("Val(Sgnl)"=T4."Status" ("Value (Signaling)")) -> ()  [unwired: 2 in, 2 out]
          }
        }
      }
      event "Dip for Protein": Value Change {
        n562 = event-data() -> ()  [unwired: 1 in, 5 out]
        n563 = case shown="True" "Dip for Protein" {
          tunnel: w889 -> [_ w891]
          tunnel: w888 -> [_ w890]
          frame False {
          }
          frame True {
            n564 = while {
              tunnel: w891 -> [w902]
              tunnel: w890 -> [w901]
              i -> [w896]
              stop <- w898 stop-if-true
              n565 = Increment(x=w896) -> (x+1=→"Dip #":i32)
              n566 = flat-sequence {
                tunnel: w901 -> [w913]
                tunnel: w902 -> [w914]
                tunnel: [w914] -> w906
                tunnel: [w913] -> w905
                tunnel: [w907] -> w892
                tunnel: [w919] -> w900
                tunnel: [w920] -> w899
                tunnel: w906 -> [w921]
                tunnel: w905 -> [w922]
                tunnel: [w917] -> w893
                tunnel: w892 -> [w917]
                tunnel: [w930] -> w904
                tunnel: w900 -> [w930]
                tunnel: [w929] -> w903
                tunnel: w899 -> [w929]
                tunnel: [w926] -> w897
                tunnel: [w925] -> w894
                tunnel: w893 -> [w925]
                tunnel: w903 -> [w950]
                tunnel: w904 -> [w951]
                tunnel: w897 -> [w952]
                tunnel: w894 -> [w949]
                tunnel: [w1008] -> w898
                frame #0 {
                  n567 = local read "Trap Pos. FB ON"() -> (w907:bool)
                  n568 = Compound Arithmetic op=AND("Flow ON\nduring dip?", "FB OFF when \nflow ON", w907) -> (w908:bool)
                  n569 = case shown="True" "Move trap \nbefore dip move?" {
                    frame False {
                    }
                    frame True {
                      n570 = property on="Trap Delta (MHz)" class="DigNum (strict)"("Val(Sgnl)"="Dipping Delta (MHz)") -> ()  [unwired: 2 in, 2 out]
                    }
                  }
                  n571 = property on="Green Laser ON/Interlacing" class="Bool (strict)"("Val(Sgnl)"="Green ON\nbefore dip?") -> ()  [unwired: 2 in, 2 out]
                  n572 = property on="Sample Channel\nFlow" class="Bool (strict)"("Val(Sgnl)"="Flow ON\nduring dip?") -> ()  [unwired: 2 in, 2 out]
                  n573 = case shown="True" w908 {
                    frame False {
                    }
                    frame True {
                      n574 = property on="Trap Pos. FB ON" class="Bool (strict)"("Val(Sgnl)"=FALSE ("Value (Signaling)")) -> ()  [unwired: 2 in, 2 out]
                    }
                  }
                }
                frame #1 {
                  n575 = local read "Saved Stage Positions"() -> (w924:dbl[][])
                  n576 = local write "Cancel dwell"(FALSE ("Cancel dwell")) -> ()
                  n577 = call "move to saved stage position.vi"("error in"=w922, "Stage VISA resource name in"=w921, "Position"="Dip Stage \nPosition", "Saved Stage Positions"=w924) -> ("VISA resource name out"=w919:refnum<visa-resource-name>, "error out"=w920:errorcluster)
                }
                frame #2 {
                  n578 = node-c288() -> (w928:T21)  [unwired: 4 in]
                  n579 = timed-loop {
                    timing: w928 -> [_]
                    timing-out: [_] -> w927
                    tunnel: [w934] -> w926
                    i -> [w931]
                    stop <- w935 stop-if-true
                    n580 = node-c288() -> ()  [unwired: 1 in, 1 out]
                    n581 = Greater Or Equal?(x=w931, y="Dip Duration (s)") -> (x >= y?=w943:bool)
                    n582 = local read "Dip for Protein"() -> (w936:bool)
                    n583 = local read "Dump Beads"() -> (w933:bool)
                    n584 = local read "Cancel dwell"() -> (w942:bool)
                    n585 = local read "Pause dwell"() -> (w939:bool)
                    n586 = Not(x=w936) -> (.not. x?=w941:bool)
                    n587 = Compound Arithmetic op=OR(w942, w943, w941) -> (w940:bool)
                    n588 = Select(t=FALSE, s=w939, f=w940) -> (s? t:f=w937:bool)
                    n589 = Not(x=w933) -> (.not. x?=w932:bool)
                    n590 = node-c288() -> ()  [unwired: 1 in, 1 out]
                    n591 = And(x=w936, y=w932) -> (x .and. y?=w934:bool)
                    n592 = Or(x=w937, y=w933) -> (x .or. y?=w935:bool)
                    "Dip Time (s)" <- w931
                  }
                  n593 = node-c288(w927) -> ()  [unwired: 1 out]
                }
                frame #3 {
                  n594 = case shown="True" w952 {
                    tunnel: w951 -> [_ w957]
                    tunnel: w950 -> [_ w956]
                    tunnel: w949 -> [_ w953]
                    frame False {
                    }
                    frame True {
                      n595 = flat-sequence {
                        tunnel: w956 -> [w961]
                        tunnel: w957 -> [w962]
                        tunnel: [w962] -> w955
                        tunnel: [w961] -> w954
                        tunnel: w953 -> [w958]
                        tunnel: w955 -> [w972]
                        tunnel: w954 -> [w971]
                        tunnel: w953 -> [w980]
                        frame #0 {
                          n596 = local read "Sample Channel\nFlow"() -> (w960:bool)
                          n597 = case shown="True" w960 {
                            tunnel: "Flow ON \nduring return\nfrom dip?" -> [w963 w966]
                            tunnel: w958 -> [_ w965]
                            frame False {
                              n598 = case shown="True" w963 {
                                frame False {
                                }
                                frame True {
                                n599 = property on="Sample Channel\nFlow" class="Bool (strict)"("Val(Sgnl)"=TRUE ("Value (Signaling)")) -> ()  [unwired: 2 in, 2 out]
                                }
                              }
                            }
                            frame True {
                              n600 = case shown="False" w966 {
                                tunnel: w965 -> [w967 _]
                                frame False {
                                n601 = property on="Trap Pos. FB ON" class="Bool (strict)"("Val(Sgnl)"=w967) -> ()  [unwired: 2 in, 2 out]
                                n602 = property on="Sample Channel\nFlow" class="Bool (strict)"("Val(Sgnl)"=FALSE ("Value (Signaling)")) -> ()  [unwired: 2 in, 2 out]
                                }
                                frame True {
                                }
                              }
                            }
                          }
                        }
                        frame #1 {
                          # "For turning on green laser before stage reaches lower spot"
                          n603 = case shown="True" "Green ON\nafter start\nreturn?" {
                            frame False {
                            }
                            frame True {
                              n604 = flat-sequence {
                                frame #0 {
                                n605 = Multiply(x="Green delay after \nstart return (s)", y=1000.0) -> (x*y=w977:dbl)
                                n606 = Wait (ms)(milliseconds to wait=w977) -> ()  [unwired: 1 out]
                                }
                                frame #1 {
                                n607 = property on="Green Laser ON/Interlacing" class="Bool (strict)"("Val(Sgnl)"=TRUE ("Value (Signaling)")) -> ()  [unwired: 2 in, 2 out]
                                }
                              }
                            }
                          }
                          n608 = local read "Saved Stage Positions"() -> (w975:dbl[][])
                          n609 = local write "Cancel dwell"(FALSE ("Cancel dwell")) -> ()
                          n610 = call "move to saved stage position.vi"("error in"=w971, "Stage VISA resource name in"=w972, "Position"="Return Stage \nPosition", "Saved Stage Positions"=w975) -> ("error out"=w973:errorcluster)  [unwired: 1 out]
                          n611 = local write "Stage Control Serial Error"(w973) -> ()
                        }
                        frame #2 {
                          n612 = property on="Trap Pos. FB ON" class="Bool (strict)"("Val(Sgnl)"=w980) -> ()  [unwired: 2 in, 2 out]
                          n613 = case shown="True" "Green ON \nafter return?" {
                            frame False {
                            }
                            frame True {
                              n614 = property on="Green Laser ON/Interlacing" class="Bool (strict)"("Val(Sgnl)"=TRUE ("Value (Signaling)")) -> ()  [unwired: 2 in, 2 out]
                            }
                          }
                          n615 = case shown="True" "Move trap after return?" {
                            frame False {
                            }
                            frame True {
                              n616 = property on="Trap Delta (MHz)" class="DigNum (strict)"("Val(Sgnl)"="Dip Trap Delta 2 (MHz)") -> ()  [unwired: 2 in, 2 out]
                            }
                          }
                          n617 = case shown="True" "Save data after return?" {
                            frame False {
                            }
                            frame True {
                              n618 = property on="Start Saving" class="Bool (strict)"("Val(Sgnl)"=TRUE ("Value (Signaling)")) -> ()  [unwired: 2 in, 2 out]
                            }
                          }
                          n619 = property on="Sample Channel\nFlow" class="Bool (strict)"("Val(Sgnl)"="Flow ON\nduring daq?") -> ()  [unwired: 2 in, 2 out]
                        }
                        frame #3 {
                          n620 = node-c288() -> (w989:T21)  [unwired: 4 in]
                          n621 = timed-loop {
                            timing: w989 -> [_]
                            timing-out: [_] -> w988
                            i -> [w990]
                            stop <- w992 stop-if-true
                            n622 = node-c288() -> ()  [unwired: 1 in, 1 out]
                            n623 = local read "Dump Beads"() -> (w991:bool)
                            n624 = Greater Or Equal?(x=w990, y="Dwell Duration (s)") -> (x >= y?=w997:bool)
                            n625 = local read "Dip for Protein"() -> (w994:bool)
                            n626 = Not(x=w994) -> (.not. x?=w993:bool)
                            n627 = Compound Arithmetic op=OR(w997, "Cancel dwell", w993) -> (w996:bool)
                            n628 = node-c288() -> ()  [unwired: 1 in, 1 out]
                            n629 = Select(t=FALSE, s="Pause dwell", f=w996) -> (s? t:f=w999:bool)
                            n630 = Or(x=w999, y=w991) -> (x .or. y?=w992:bool)
                            "Dwell Time (s)" <- w990
                          }
                          n631 = node-c288(w988) -> ()  [unwired: 1 out]
                        }
                      }
                    }
                  }
                }
                frame #4 {
                  n632 = local read "Dip for Protein"() -> (w1009:bool)
                  n633 = local read "Dump Beads"() -> (w1006:bool)
                  n634 = local write "Cancel dwell"(FALSE ("Cancel dwell")) -> ()
                  n635 = Not(x=w1009) -> (.not. x?=w1010:bool)
                  n636 = Not(x="Cont. Repeat Dipping?") -> (.not. x?=w1012:bool)
                  n637 = Compound Arithmetic op=OR(w1010, w1012, w1006) -> (w1008:bool)
                }
              }
            }
          }
        }
      }
      event "Profile": Value Change {
        n638 = event-data() -> ()  [unwired: 1 in, 5 out]
        n639 = flat-sequence {
          tunnel: w1021 -> [w1024]
          tunnel: w1020 -> [w1032]
          tunnel: [w1026] -> w1019
          tunnel: [w1025] -> w1018
          tunnel: [w1023] -> w1016
          tunnel: [w1022] -> w1013
          tunnel: w1019 -> [w1039]
          tunnel: w1018 -> [w1038]
          tunnel: [w1036] -> w1017
          tunnel: w1016 -> [w1037]
          tunnel: [w1035] -> w1015
          tunnel: [w1034] -> w1014
          tunnel: w1013 -> [w1034]
          tunnel: w1017 -> [w1043]
          tunnel: w1015 -> [w1042]
          tunnel: w1014 -> [w1041]
          frame #0 {
            n640 = call "Read Stage Position.vi"("error in"=w1032, "VISA resource name in"=w1024) -> ("Current Position"=w1022:cluster{dbl, dbl, dbl}, "error out"=w1025:errorcluster, "VISA resource name out"=w1023:refnum<visa-resource-name>)  [unwired: 1 out]
            "Current Position" <- w1022
            n641 = local write "Stage Control Serial Error"(w1025) -> ()
            n642 = Unbundle(w1022) -> (w1029:dbl, w1031:dbl, w1027:dbl)
            n643 = Add(x=w1031, y="Y change (mm)") -> (x+y=w1028:dbl)
            n644 = Bundle(w1029, w1028, w1027) -> (w1026:cluster{dbl, dbl, dbl})  [unwired: 1 in]
          }
          frame #1 {
            # "move to new position and start saving"
            n645 = local write "Stage Moving"(TRUE ("Stage Moving")) -> ()
            n646 = local write "Start Saving"(TRUE ("Start Saving")) -> ()
            n647 = call "Set Stage Position.vi"("Position"=w1039, "error in"=w1038, "VISA resource name in"=w1037) -> ("error out"=w1035:errorcluster, "VISA resource name out"=w1036:refnum<visa-resource-name>)  [unwired: 1 out]
          }
          frame #2 {
            # "go back to start"
            n648 = call "Set Stage Position.vi"("Position"=w1041, "error in"=w1042, "VISA resource name in"=w1043) -> ()  [unwired: 3 out]
          }
          frame #3 {
            # "stop saving"
            n649 = local write "Stop Saving"(TRUE ("Stop Saving")) -> ()
            n650 = local write "Stage Moving"(FALSE ("Stage Moving")) -> ()
          }
        }
      }
      event "Move to Position 1", "Move to Position 2", "Move to Position 3", "Move to Position 4", "Move to Position 5", "Lower Ch. Cap.": Value Change {
        n651 = event-data() -> ()  [unwired: 1 in, 5 out]
        n652 = Or(x="Move to Position 5", y="Lower Ch. Cap.") -> (x .or. y?=w1049:bool)
        n653 = Build Array("Move to Position 1", "Move to Position 2", "Move to Position 3", "Move to Position 4", w1049) -> (w1052:bool[])
        n654 = Boolean Array To Number(Boolean array=w1052) -> (number=w1051:u32)
        n655 = Logarithm Base 2(1:w1051) -> (0:w1050:dbl)
        n656 = flat-sequence {
          tunnel: w1050 -> [w1061]
          tunnel: w1047 -> [w1059]
          tunnel: w1046 -> [w1058]
          frame #0 {
            n657 = local read "Saved Stage Positions"() -> (w1069:dbl[][])
            n658 = Array Subset(array=w1069, index (row)=w1061, length (row)=1 ("length"), index (col)=1 ("index"), length (col)=3 ("length")) -> (w1066:dbl[][])
            n659 = Reshape Array(w1066, 3 ("dimension size")) -> (w1064:dbl[])
            n660 = Array To Cluster(array=w1064) -> (cluster=w1063:cluster{"[0]":dbl, "[1]":dbl, "[2]":dbl})
            n661 = call "Set Stage Position.vi"("Position"=w1063, "error in"=w1058, "VISA resource name in"=w1059) -> ("error out"=w1062:errorcluster)  [unwired: 2 out]
            n662 = local write "Stage Moving"(TRUE ("Stage Moving")) -> ()
            n663 = local write "Stage Control Serial Error"(w1062) -> ()
          }
          frame #1 {
            n664 = local write "Stage Moving"(FALSE ("Stage Moving")) -> ()
            n665 = call <vilib>:"Beep.vi"() -> ()  [unwired: 3 in, 9 out]
          }
        }
      }
      event "Got ADig bead": Value Change {
        n666 = event-data() -> ()  [unwired: 1 in, 5 out]
        n667 = flat-sequence {
          frame #0 {
            n668 = local read "Cap 1 Samp Flow ON"() -> (w1073:bool)
            n669 = case shown="True" w1073 {
              frame False {
              }
              frame True {
                n670 = property on="Sample Channel\nFlow" class="Bool (strict)"("Val(Sgnl)"=TRUE ("Value (Signaling)")) -> ()  [unwired: 2 in, 2 out]
              }
            }
          }
          frame #1 {
            n671 = property on="Inject Pump 3" class="Bool (strict)"("Val(Sgnl)"=FALSE ("Value (Signaling)")) -> ()  [unwired: 2 in, 2 out]
          }
          frame #2 {
            n672 = property on="Move Cap. 1 (DNA Bottom)" class="Bool (strict)"("Val(Sgnl)"=TRUE ("Value (Signaling)")) -> ()  [unwired: 2 in, 2 out]
          }
        }
      }
      event "Force FB Data\nScript": Value Change {
        n673 = event-data() -> ()  [unwired: 1 in, 5 out]
        n674 = flat-sequence {
          tunnel: w1082 -> [w1086]
          tunnel: w1083 -> [w1087]
          tunnel: [w1087] -> w1078
          tunnel: [w1086] -> w1077
          tunnel: w1078 -> [w1090]
          tunnel: w1077 -> [w1089]
          tunnel: ["Trap Trig Fl."] -> w1079
          tunnel: [w1115] -> w1080
          tunnel: w1079 -> [w1115]
          tunnel: [w1119] -> w1081
          tunnel: w1080 -> [w1119]
          tunnel: w1081 -> [w1121]
          frame #0 {
            n675 = property on="Trap Delta (MHz)" class="DigNum (strict)"("Val(Sgnl)"="Trap Delta Before Moving") -> ()  [unwired: 2 in, 2 out]
          }
          frame #1 {
            n676 = local read "Saved Stage Positions"() -> (w1092:dbl[][])
            n677 = local write "FB Trap Pos Offset"(0.0 ("FB Trap Pos Offset")) -> ()
            n678 = property on="Trap Pos. FB Offset Factor" class="DigNum (strict)"("Val(Sgnl)"=i64 0 ("Value (Signaling)")) -> ()  [unwired: 2 in, 2 out]
            n679 = local write "Stage Moving"(TRUE ("Stage Moving")) -> ()
